vi "DoubleToString.vi"(5 "SignificantDigits (8)":u32=8, 7 "Format (SI notation)":T1(ring)=enum."SI notation", 11 "Double":dbl) -> (3 "String":string)   [LabVIEW 2013, in "VariableManagerAPI.lvlib"]
doc: "Format double precision number to a string.\n\nFormat:\n1. Floating point - number in decimal point notation\n2. Scienctific SI - number with exponent multiple of 3\n3. Automatic SI - automatically chose format 1 or 2\n4. SI notation - number with SI prefix\n\nSignificantDigits value range is [1,15]"
uses:
  VariableManagerAPI.lvlib
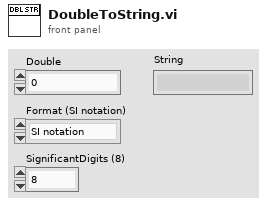
[diagram p1: front panel]
types:
  T1 = enum16{"Floating point", "Scientific SI", "Automatic SI", "SI notation"}
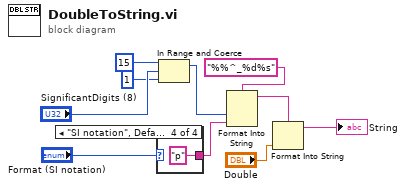
[diagram p0: block diagram]
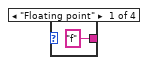
[diagram p2: hidden frame]
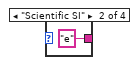
[diagram p3: hidden frame]
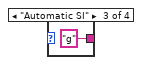
[diagram p4: hidden frame]
diagram:
  n1 = case shown="\"SI notation\", Default" "Format (SI notation)" {
    tunnel: ["f" "e" "g" "p"] -> w8
    frame "Floating point" {
    }
    frame "Scientific SI" {
    }
    frame "Automatic SI" {
    }
    frame "SI notation", Default {
    }
  }
  n2 = In Range and Coerce(upper limit=u32 15 ("lower limit"), x="SignificantDigits (8)", lower limit=u32 1) -> (coerced(x)=w3:u32)  [unwired: 1 out]
  n3 = Format Into String(format string="%%^_%d%s", w3, w8) -> (resulting string=w7:string)  [unwired: 2 in, 1 out]
  n4 = Format Into String(format string=w7, "Double") -> (resulting string=→"String":string)  [unwired: 2 in, 1 out]
